vi "EMBL Objective Lock.vi"() -> ()   [LabVIEW 2016]
uses:
  Hardware Configuration/Hardware Configuration Controls/Device Type.ctl
  Hardware Configuration/Hardware Configuration Controls/Device Function.ctl
  Device Library/Cameras/IDS/IDS Controls/IDS Actions.ctl
  Device Library/Stages/Stages Controls/Stage Actions.ctl
  <vilib>/addons/control/pid/pid.llb/PID (DBL Array).vi
  <vilib>/addons/control/pid/NI_PID_pid.lvlib
panel:
  in  "Invert Y":bool
  in  "Invert X":bool
  in  "Flip XY":bool=TRUE
  out "Z Moving":bool
  out "XY Moving":bool
  in  "Lock Z":bool
  in  "Lock Obectives":bool
  in  "Set Lock Position":bool
  in  "Frames Accums":u16=10
  out "Lock Position":dbl[](array[numeric])=[25.486084426867002, 23.515775149080227, -0.6325794284348785]
  out "Current XYZ Positions":dbl[](array[numeric])=[25.44687943773384, 23.028592568780166, -0.15399804743769252]
  out "Difference":dbl[](array[numeric])=[-1.1037470842083863, -0.0443794761167986, 0.0]
  out "Drift Detected":bool
  in  "Z Tolorence":dbl=0.1 format="%#_6f"
  in  "XY Tolorence":dbl=0.1
  out "Z Position":dbl(graph)=-0.15399804743769252
  in  "Display time (ms)":u32=20
  out "Refresh rate":dbl=1.996007984031936
  out "XY Positions":cluster{dbl, dbl}(graph)={25.44687943773384, 23.028592568780166}
  out "ROI":u16[][](graph)=[[103, 104, 97, 86, 80, 79, 59, 70, 55, 56, 44, 54, 47, 62, 70, 96, 116, 143, 146, 167, 194, 216, 232, 243, 276, 307, 316, 310, 318, 306, 280, 274, 267, 251, 222, 199, 175, 157, 125, 107, 87, 79, 57, 56, 38, 36, 28, 30, 24, 26], [123, 104, 98, 92, 87, 76, 65, 64, 66, 52, 69, 62, 71, 73, 96, 114, 138, 166, 199, 194, 218, 242, 260, 295, 331, 342, 361, 346, 350, 340, 317, 299, 293, 261, 252, 217, 194, 165, 145, 128, 105, 87, 76, 51, 48, 30, 28, 22, 28, 24], [122, 120, 100, 101, 92, 83, 72, 80, 72, 75, 78, 75, 87, 106, 115, 133, 161, 204, 233, 237, 264, 308, 326, 347, 361, 372, 377, 375, 398, 398, 373, 345, 325, 304, 289, 250, 222, 195, 169, 151, 119, 94, 76, 64, 40, 34, 26, 22, 20, 40], [145, 128, 110, 114, 100, 92, 88, 78, 84, 89, 95, 101, 121, 132, 142, 159, 213, 251, 284, 298, 327, 380, 398, 409, 441, 433, 455, 453, 443, 443, 422, 397, 394, 352, 342, 288, 269, 231, 203, 175, 145, 113, 98, 62, 57, 38, 39, 28, 36, 39], [139, 139, 120, 127, 99, 110, 95, 101, 109, 110, 107, 129, 145, 174, 180, 217, 248, 292, 318, 359, 384, 454, 490, 490, 525, 519, 514, 518, 526, 513, 506, 478, 441, 413, 379, 338, 301, 269, 233, 202, 155, 129, 104, 79, 54, 52, 38, 34, 33, 32], [163, 150, 138, 123, 119, 123, 121, 106, 133, 139, 152, 156, 181, 200, 223, 260, 317, 350, 367, 397, 455, 527, 570, 568, 603, 588, 628, 616, 635, 622, 594, 550, 534, 480, 451, 387, 350, 312, 264, 215, 187, 145, 125, 93, 78, 57, 44, 45, 40, 34], [167, 162, 159, 145, 130, 141, 127, 137, 147, 161, 172, 202, 214, 237, 271, 330, 391, 414, 453, 471, 518, 611, 636, 655, 673, 706, 747, 724, 736, 729, 670, 633, 619, 550, 509, 458, 389, 342, 288, 252, 199, 172, 145, 117, 98, 78, 59, 53, 44, 46], [189, 174, 175, 161, 162, 150, 154, 165, 176, 192, 217, 254, 269, 282, 330, 382, 460, 502, 550, 586, 631, 694, 719, 759, 772, 816, 837, 848, 825, 831, 774, 709, 675, 607, 560, 490, 454, 380, 334, 280, 241, 200, 165, 133, 117, 87, 72, 62, 58, 56], [189, 194, 182, 181, 174, 173, 171, 197, 200, 212, 243, 300, 316, 352, 386, 460, 509, 577, 651, 704, 737, 784, 823, 844, 891, 920, 949, 942, 941, 922, 849, 810, 743, 672, 617, 545, 500, 436, 383, 336, 276, 243, 195, 159, 129, 117, 91, 85, 70, 67], [212, 214, 200, 185, 208, 193, 200, 218, 239, 254, 305, 348, 365, 409, 482, 511, 595, 660, 739, 790, 846, 925, 944, 985, 1009, 1050, 1073, 1057, 1035, 1038, 958, 864, 842, 773, 705, 631, 589, 518, 444, 385, 312, 261, 231, 181, 167, 132, 114, 105, 93, 78], [217, 227, 216, 221, 229, 216, 224, 260, 270, 310, 355, 382, 414, 478, 553, 613, 668, 765, 847, 907, 965, 1016, 1068, 1109, 1144, 1210, 1225, 1196, 1155, 1130, 1084, 1019, 966, 875, 836, 732, 645, 589, 505, 449, 365, 309, 253, 213, 183, 157, 133, 132, 102, 101], [238, 243, 222, 231, 239, 247, 267, 294, 308, 358, 414, 446, 479, 541, 622, 689, 811, 874, 960, 1009, 1044, 1134, 1223, 1235, 1341, 1337, 1371, 1347, 1340, 1318, 1197, 1152, 1049, 986, 950, 818, 749, 636, 571, 490, 413, 357, 306, 248, 213, 179, 155, 144, 137, 113], [255, 255, 243, 253, 247, 265, 299, 330, 343, 398, 467, 506, 544, 628, 709, 808, 881, 971, 1090, 1152, 1188, 1262, 1309, 1366, 1443, 1501, 1426, 1450, 1425, 1386, 1315, 1221, 1199, 1102, 1011, 902, 816, 728, 642, 554, 484, 410, 354, 297, 252, 222, 178, 165, 154, 143], [256, 252, 253, 273, 281, 290, 340, 355, 389, 439, 517, 547, 608, 697, 814, 877, 967, 1099, 1208, 1299, 1324, 1416, 1427, 1531, 1599, 1607, 1620, 1563, 1556, 1493, 1437, 1362, 1277, 1187, 1093, 991, 922, 815, 721, 627, 541, 490, 386, 338, 282, 241, 222, 197, 187, 160], [269, 283, 273, 300, 302, 316, 365, 389, 441, 506, 554, 594, 684, 794, 899, 995, 1052, 1168, 1286, 1349, 1448, 1558, 1587, 1670, 1742, 1762, 1719, 1716, 1679, 1597, 1517, 1449, 1429, 1313, 1239, 1096, 985, 938, 800, 705, 603, 518, 442, 379, 329, 283, 244, 234, 203, 197], [290, 293, 287, 314, 322, 353, 404, 423, 476, 538, 607, 643, 714, 841, 980, 1084, 1190, 1288, 1381, 1496, 1596, 1625, 1712, 1802, 1901, 1923, 1864, 1865, 1796, 1795, 1654, 1567, 1540, 1396, 1346, 1218, 1132, 957, 879, 773, 667, 577, 492, 418, 352, 307, 274, 243, 241, 211], [295, 310, 309, 343, 344, 381, 431, 475, 505, 566, 667, 706, 793, 914, 1042, 1173, 1301, 1388, 1502, 1657, 1693, 1753, 1789, 1942, 1994, 2031, 1984, 2006, 1939, 1872, 1762, 1653, 1593, 1497, 1410, 1262, 1165, 1022, 927, 813, 683, 632, 545, 452, 391, 356, 296, 272, 253, 243], [322, 320, 327, 356, 370, 408, 458, 505, 547, 596, 680, 732, 874, 1003, 1103, 1207, 1342, 1466, 1617, 1729, 1812, 1865, 1945, 2030, 2069, 2048, 2066, 2075, 2044, 1935, 1828, 1739, 1715, 1563, 1495, 1327, 1214, 1118, 990, 889, 773, 665, 565, 492, 429, 384, 336, 318, 282, 264], [322, 340, 336, 379, 396, 427, 466, 526, 551, 655, 717, 786, 913, 1093, 1189, 1285, 1394, 1566, 1699, 1814, 1892, 1998, 2065, 2147, 2195, 2182, 2206, 2162, 2124, 2065, 1962, 1865, 1793, 1645, 1595, 1427, 1305, 1175, 1051, 909, 810, 690, 603, 545, 456, 408, 366, 333, 308, 281], [332, 343, 355, 389, 409, 441, 487, 506, 576, 658, 778, 849, 966, 1129, 1229, 1342, 1478, 1619, 1781, 1865, 1942, 2021, 2128, 2217, 2270, 2295, 2300, 2280, 2154, 2146, 2027, 1923, 1855, 1712, 1638, 1482, 1338, 1197, 1086, 941, 845, 736, 646, 554, 500, 431, 397, 353, 352, 305], [324, 350, 352, 394, 420, 441, 499, 537, 589, 697, 802, 898, 1009, 1146, 1310, 1345, 1516, 1664, 1848, 1994, 2007, 2120, 2204, 2269, 2301, 2343, 2347, 2332, 2272, 2219, 2085, 1970, 1880, 1743, 1687, 1477, 1341, 1240, 1140, 990, 870, 758, 658, 593, 519, 465, 421, 385, 364, 327], [325, 344, 347, 388, 405, 426, 494, 552, 618, 707, 828, 939, 1040, 1173, 1323, 1412, 1570, 1699, 1839, 2004, 2077, 2157, 2294, 2290, 2367, 2359, 2417, 2368, 2293, 2208, 2118, 2025, 1924, 1825, 1699, 1533, 1389, 1265, 1132, 1020, 905, 799, 696, 610, 548, 490, 460, 411, 385, 343], [300, 328, 326, 366, 391, 426, 476, 562, 625, 723, 864, 938, 1026, 1145, 1342, 1501, 1578, 1748, 1866, 2015, 2089, 2226, 2252, 2306, 2387, 2414, 2428, 2400, 2367, 2264, 2171, 2050, 1955, 1810, 1736, 1557, 1428, 1274, 1175, 1043, 918, 824, 708, 662, 571, 524, 461, 435, 381, 355], [293, 311, 331, 349, 383, 420, 499, 591, 644, 722, 849, 930, 1049, 1146, 1345, 1497, 1633, 1704, 1926, 2019, 2153, 2262, 2232, 2313, 2410, 2386, 2460, 2393, 2372, 2289, 2132, 2046, 1917, 1802, 1696, 1551, 1444, 1278, 1201, 1067, 947, 839, 743, 663, 596, 520, 486, 434, 400, 369], [289, 304, 321, 348, 398, 425, 484, 574, 643, 723, 815, 928, 1041, 1168, 1352, 1492, 1629, 1716, 1871, 2033, 2144, 2270, 2274, 2282, 2393, 2320, 2396, 2393, 2377, 2243, 2173, 2010, 1928, 1828, 1686, 1553, 1444, 1313, 1201, 1040, 924, 863, 759, 668, 610, 560, 495, 456, 418, 365], [289, 300, 333, 340, 393, 417, 476, 550, 624, 683, 803, 907, 1022, 1146, 1343, 1474, 1614, 1698, 1823, 1980, 2060, 2168, 2226, 2345, 2332, 2306, 2376, 2439, 2349, 2280, 2206, 2034, 1930, 1797, 1720, 1542, 1425, 1264, 1175, 1031, 949, 847, 759, 673, 594, 552, 504, 452, 406, 380], [278, 302, 314, 331, 358, 417, 458, 514, 584, 655, 765, 914, 1051, 1127, 1277, 1411, 1589, 1717, 1824, 1958, 2060, 2168, 2226, 2248, 2274, 2208, 2320, 2285, 2217, 2187, 2117, 2022, 1907, 1782, 1668, 1489, 1388, 1257, 1166, 1021, 936, 831, 756, 678, 617, 567, 497, 446, 412, 381], [263, 263, 284, 309, 337, 386, 416, 478, 561, 657, 765, 891, 1016, 1109, 1230, 1350, 1538, 1647, 1755, 1867, 1998, 2119, 2201, 2171, 2217, 2220, 2252, 2205, 2185, 2145, 2031, 1937, 1861, 1722, 1666, 1449, 1372, 1251, 1122, 1021, 914, 825, 753, 649, 601, 541, 480, 433, 414, 371], [226, 235, 264, 284, 305, 362, 413, 459, 551, 648, 727, 828, 965, 1084, 1188, 1337, 1498, 1606, 1700, 1782, 1912, 2021, 2109, 2097, 2187, 2116, 2153, 2099, 2116, 2030, 1952, 1824, 1797, 1640, 1555, 1427, 1315, 1204, 1102, 1012, 874, 803, 725, 642, 583, 513, 469, 434, 399, 389], [219, 215, 243, 261, 285, 338, 392, 432, 532, 627, 703, 785, 898, 1017, 1134, 1267, 1418, 1497, 1634, 1742, 1811, 1953, 1954, 2040, 2103, 2065, 2018, 2004, 1961, 1902, 1821, 1756, 1680, 1558, 1491, 1351, 1265, 1124, 1040, 962, 823, 760, 658, 605, 543, 506, 428, 425, 413, 395], [202, 211, 218, 257, 275, 323, 381, 419, 472, 570, 633, 700, 837, 1004, 1109, 1197, 1344, 1444, 1568, 1669, 1677, 1827, 1871, 1959, 2000, 1944, 1967, 1902, 1845, 1803, 1716, 1664, 1575, 1448, 1358, 1227, 1157, 1052, 953, 864, 759, 709, 623, 547, 510, 472, 447, 427, 416, 380], [188, 196, 201, 233, 253, 272, 321, 371, 426, 502, 616, 698, 788, 932, 1046, 1105, 1220, 1334, 1449, 1565, 1618, 1702, 1739, 1796, 1845, 1875, 1858, 1759, 1739, 1708, 1614, 1500, 1458, 1320, 1294, 1141, 1051, 962, 884, 789, 702, 652, 576, 527, 500, 443, 434, 421, 405, 363], [158, 174, 181, 201, 213, 242, 283, 339, 395, 485, 570, 658, 745, 835, 944, 1063, 1148, 1258, 1373, 1465, 1518, 1620, 1634, 1653, 1707, 1751, 1725, 1652, 1627, 1600, 1476, 1400, 1346, 1214, 1165, 1021, 973, 885, 797, 739, 665, 608, 540, 517, 466, 442, 398, 393, 383, 339], [134, 139, 149, 164, 196, 216, 269, 326, 372, 436, 512, 601, 681, 726, 876, 1004, 1081, 1152, 1240, 1336, 1439, 1485, 1522, 1523, 1582, 1548, 1573, 1576, 1518, 1482, 1381, 1311, 1212, 1146, 1083, 968, 891, 794, 748, 670, 617, 567, 508, 466, 454, 409, 375, 359, 345, 332], [125, 123, 139, 146, 169, 212, 223, 283, 332, 374, 440, 524, 614, 701, 790, 902, 1003, 1052, 1133, 1233, 1307, 1359, 1414, 1423, 1432, 1411, 1404, 1415, 1393, 1349, 1304, 1217, 1147, 1021, 991, 882, 819, 764, 676, 625, 569, 519, 460, 433, 410, 370, 334, 334, 312, 318], [111, 107, 130, 126, 151, 171, 197, 236, 290, 340, 388, 462, 570, 637, 718, 789, 895, 921, 1044, 1081, 1153, 1221, 1285, 1299, 1316, 1261, 1289, 1261, 1220, 1218, 1133, 1065, 1026, 955, 883, 821, 747, 662, 627, 554, 523, 474, 421, 386, 373, 338, 326, 316, 318, 293], [94, 95, 90, 117, 116, 148, 167, 199, 254, 314, 359, 414, 503, 563, 646, 677, 797, 879, 963, 999, 1028, 1119, 1123, 1174, 1195, 1203, 1143, 1103, 1071, 1052, 1005, 938, 891, 842, 780, 699, 650, 569, 529, 500, 446, 400, 367, 344, 316, 298, 300, 298, 313, 288], [75, 70, 72, 92, 101, 114, 161, 189, 226, 264, 326, 361, 426, 492, 598, 631, 689, 775, 822, 907, 922, 977, 984, 1025, 1053, 1064, 1043, 994, 966, 927, 860, 813, 778, 688, 663, 589, 547, 497, 446, 407, 374, 339, 324, 309, 300, 285, 294, 283, 284, 272], [62, 73, 60, 85, 85, 111, 129, 161, 180, 221, 268, 326, 369, 425, 506, 577, 604, 657, 736, 830, 823, 867, 877, 899, 906, 892, 907, 883, 853, 838, 772, 719, 677, 615, 572, 529, 487, 430, 399, 369, 340, 314, 298, 288, 267, 263, 272, 248, 243, 248], [61, 54, 50, 60, 74, 81, 97, 124, 158, 186, 230, 287, 342, 365, 427, 479, 549, 582, 617, 695, 711, 746, 804, 776, 794, 796, 763, 753, 743, 723, 678, 640, 604, 539, 519, 462, 409, 381, 345, 325, 288, 274, 254, 249, 245, 230, 221, 226, 229, 233], [42, 41, 40, 48, 54, 72, 79, 105, 145, 165, 195, 243, 272, 321, 351, 419, 473, 530, 540, 587, 617, 674, 683, 697, 698, 661, 648, 646, 608, 593, 573, 535, 506, 463, 438, 381, 358, 326, 290, 278, 249, 237, 225, 209, 205, 197, 196, 209, 220, 224], [44, 36, 36, 32, 46, 52, 77, 88, 107, 144, 164, 186, 237, 283, 317, 347, 389, 434, 487, 525, 507, 548, 565, 604, 610, 574, 557, 566, 527, 496, 477, 443, 401, 376, 340, 317, 287, 259, 241, 216, 208, 188, 181, 175, 178, 182, 190, 198, 194, 206], [29, 39, 34, 37, 30, 42, 64, 69, 87, 117, 147, 173, 195, 239, 282, 301, 331, 375, 412, 454, 458, 478, 488, 491, 494, 479, 488, 480, 461, 425, 393, 370, 330, 305, 287, 251, 226, 208, 194, 175, 165, 167, 158, 165, 162, 171, 165, 175, 175, 178], [38, 20, 22, 26, 34, 30, 48, 60, 88, 95, 125, 145, 170, 188, 233, 271, 303, 313, 338, 368, 398, 399, 422, 405, 408, 406, 401, 390, 383, 366, 335, 308, 290, 257, 242, 210, 192, 173, 167, 146, 150, 136, 139, 137, 146, 140, 152, 159, 152, 158], [36, 24, 25, 23, 20, 39, 36, 56, 68, 87, 89, 118, 145, 170, 191, 221, 250, 277, 285, 317, 320, 350, 355, 351, 360, 331, 319, 315, 292, 279, 268, 249, 235, 205, 190, 176, 154, 141, 132, 116, 117, 127, 115, 118, 117, 125, 126, 141, 145, 159], [24, 23, 28, 22, 24, 26, 31, 39, 50, 67, 81, 95, 135, 154, 173, 180, 209, 233, 248, 257, 270, 286, 289, 302, 297, 284, 278, 258, 237, 219, 202, 178, 175, 156, 149, 129, 118, 107, 102, 87, 91, 96, 94, 94, 106, 116, 126, 130, 138, 135], [20, 28, 26, 26, 27, 20, 38, 48, 50, 69, 84, 90, 102, 118, 146, 169, 179, 204, 208, 240, 234, 255, 239, 230, 237, 237, 232, 223, 202, 196, 171, 155, 133, 129, 108, 102, 90, 84, 75, 78, 78, 84, 84, 100, 101, 108, 100, 109, 109, 122], [26, 27, 29, 30, 26, 20, 40, 46, 54, 50, 66, 86, 96, 113, 133, 151, 173, 167, 177, 184, 219, 219, 203, 201, 199, 180, 180, 170, 159, 152, 139, 119, 106, 93, 93, 81, 75, 62, 70, 64, 74, 64, 82, 74, 86, 90, 91, 100, 107, 112], [22, 23, 25, 25, 21, 32, 34, 34, 40, 50, 60, 72, 92, 102, 111, 129, 140, 164, 161, 165, 163, 187, 180, 182, 165, 159, 151, 141, 124, 114, 100, 103, 84, 81, 70, 63, 54, 57, 49, 55, 52, 52, 58, 60, 75, 81, 81, 100, 94, 106], [36, 25, 25, 20, 30, 20, 34, 42, 52, 55, 69, 71, 88, 92, 114, 111, 127, 126, 146, 154, 158, 148, 148, 145, 150, 143, 129, 115, 113, 90, 88, 64, 66, 50, 47, 40, 43, 42, 48, 39, 48, 52, 54, 68, 69, 77, 80, 82, 86, 80]]
  in  "ROI Half Width":i32=25
  out "Intensity Graph":u16[][](graph)
  in  "Quit":bool
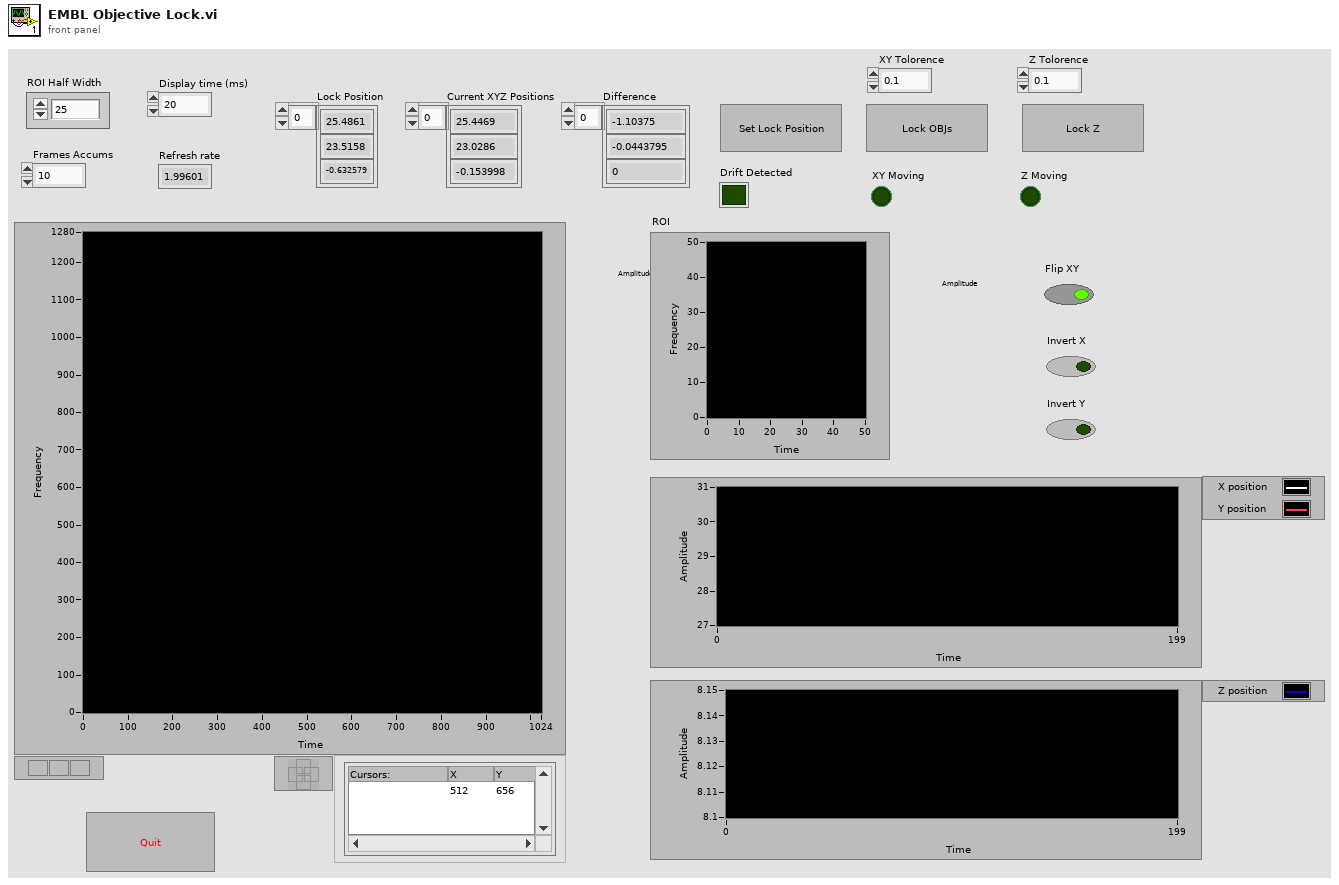
[diagram p1: front panel]
types:
  T1 = typedef "Stage Actions.ctl" = enum16{"Get Position", "MVR", "MOVE", "HALT", "ONTARGET", "ERROR", "REFERENCE", "INIT", "VELOCITY", "STATUS", "EXIT", "HOME", "ZEROPOS", "NANOPOS", "ANALOG", "QUIT"}
  T2 = typedef "IDS Actions.ctl" = enum16{"Error Check", "Initialize", "Preview", "Record", "Abort", "Record Settings", "Set Parameter", "Get Parameter", "Set ROI", "Get ROI", "Status", "Quit"}
  T3 = typedef "Device Function.ctl" = enum16{"Primary", "Secondary", "Overview", "Wide Field Drift Correction", "642 nm Excitation", "560 nm Excitation", "546 nm Excitation", "488 nm Excitation", "405 nm Excitation", "Objective Drift Correction", "4Pi Objective Lock", "Objective XY", "Objective Z", "Sample XY", "Sample Coarse Z", "Sample Z", "4Pi Lower", "4Pi Upper", "Adj Cavity", "Line Scanning", "Alert"}
  T4 = typedef "Device Type.ctl" = enum16{"AOTF", "Camera", "Deformable Mirror", "Laser", "Shutter", "Stage", "Waveform", "Email"}
  T5 = cluster{"proportional gain (Kc)":dbl, "integral time (Ti, min)":dbl, "derivative time (Td, min)":dbl}[]
  T6 = typedef "LVCursorListTypeDef.ctl" = cluster{"Name":string, "Color":u32, "Style":u8, "Point Style":u8, "Name Visible":bool, "Allow Drag":bool, "Cursor Mode":u32, "Plot":i32, "Index":i32, "Position":cluster{"X":dbl, "Y":dbl}, "X Scale":u32, "Y Scale":u32, "Watch Plots":i32[], "Watch All Plots":bool, "Plot Area":i32, "Label Offset":cluster{"X":dbl, "Y":dbl}}[]
  T7 = cluster{"Name":string, "Color":u32, "Style":u8, "Point Style":u8, "Name Visible":bool, "Allow Drag":bool, "Cursor Mode":u32, "Plot":i32, "Index":i32, "Position":cluster{"X":dbl, "Y":dbl}, "X Scale":u32, "Y Scale":u32, "Watch Plots":i32[], "Watch All Plots":bool, "Plot Area":i32, "Label Offset":cluster{"X":dbl, "Y":dbl}}
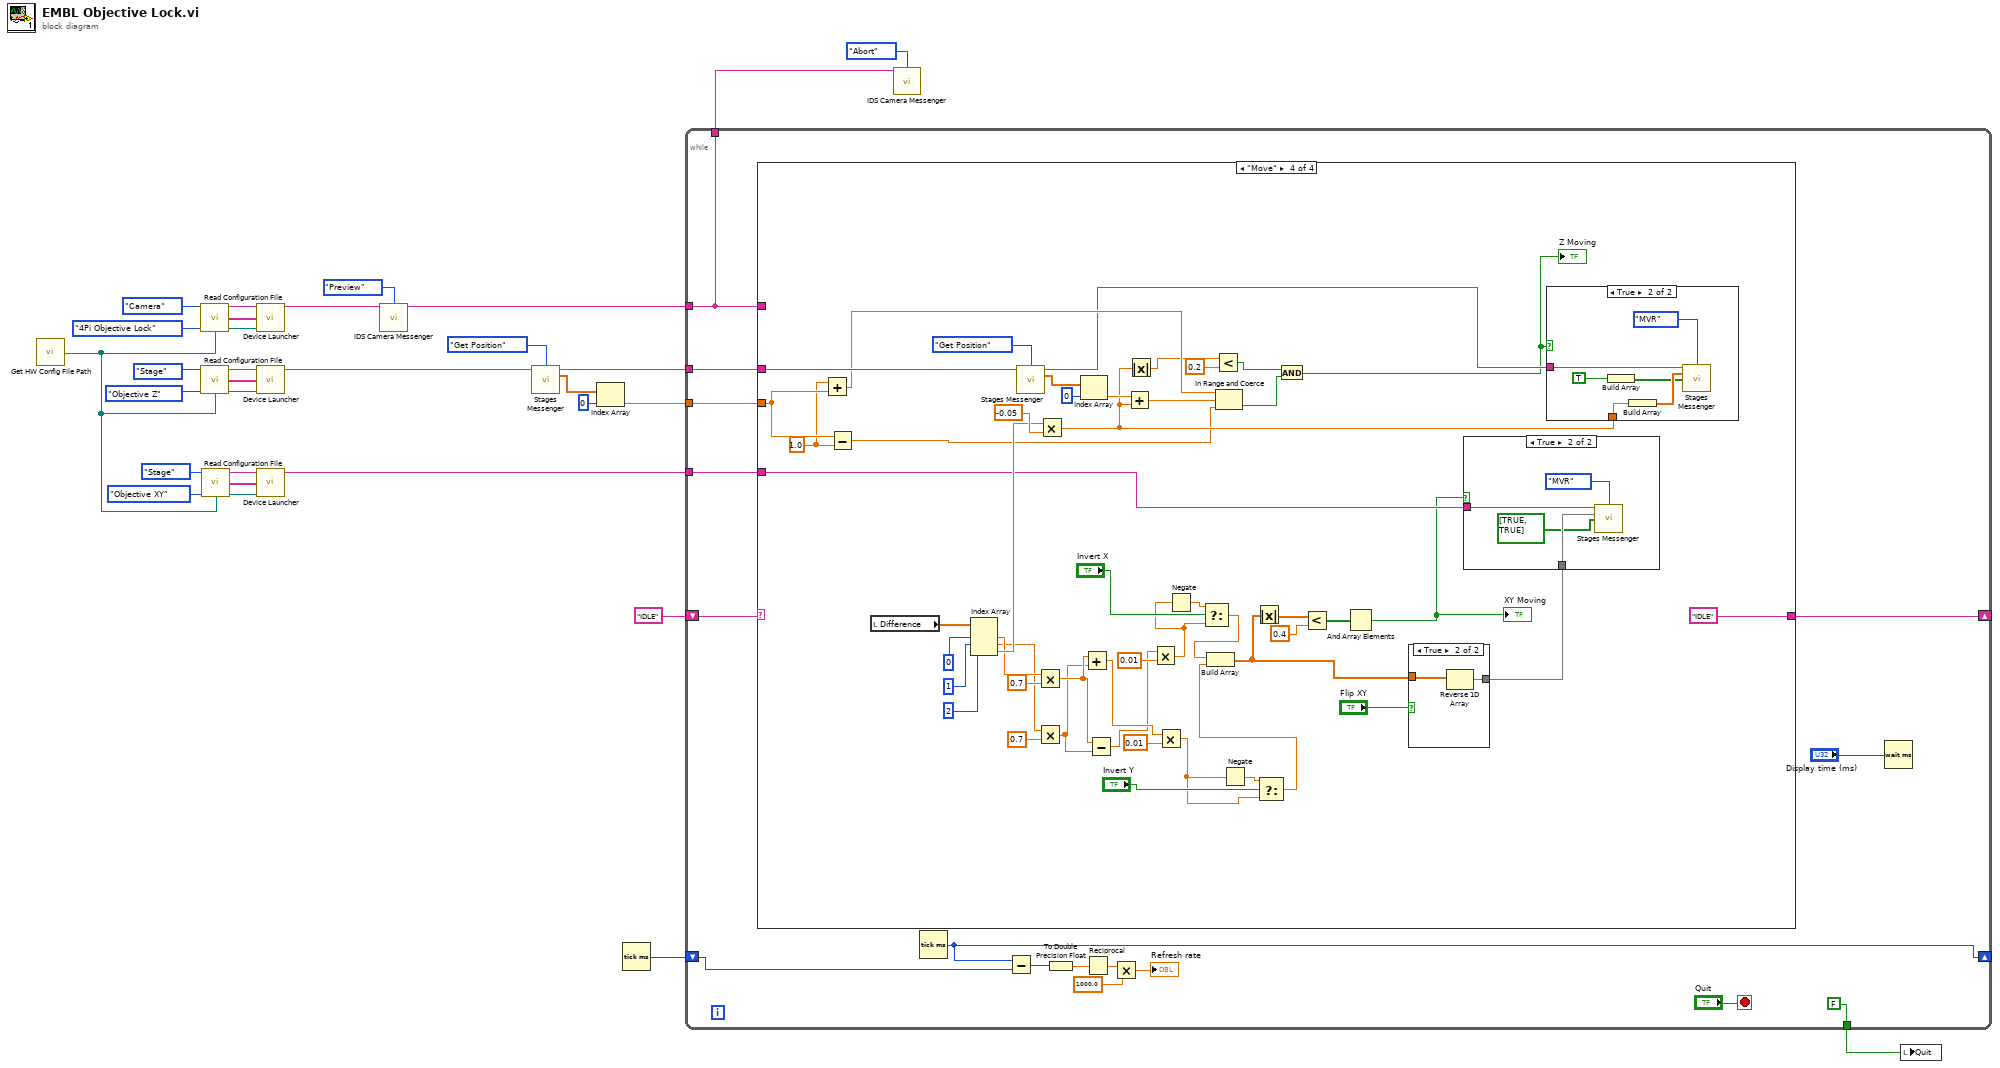
[diagram p0: block diagram]
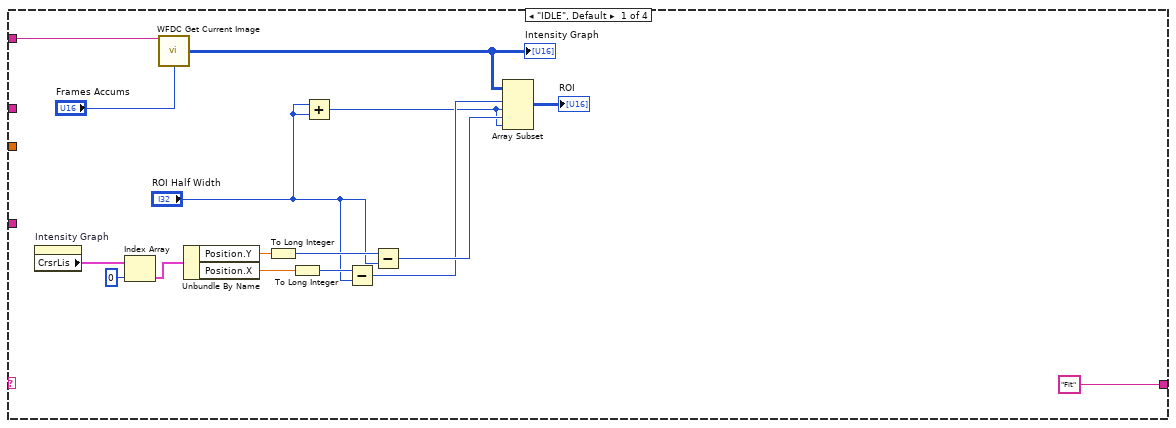
[diagram p2: hidden frame]
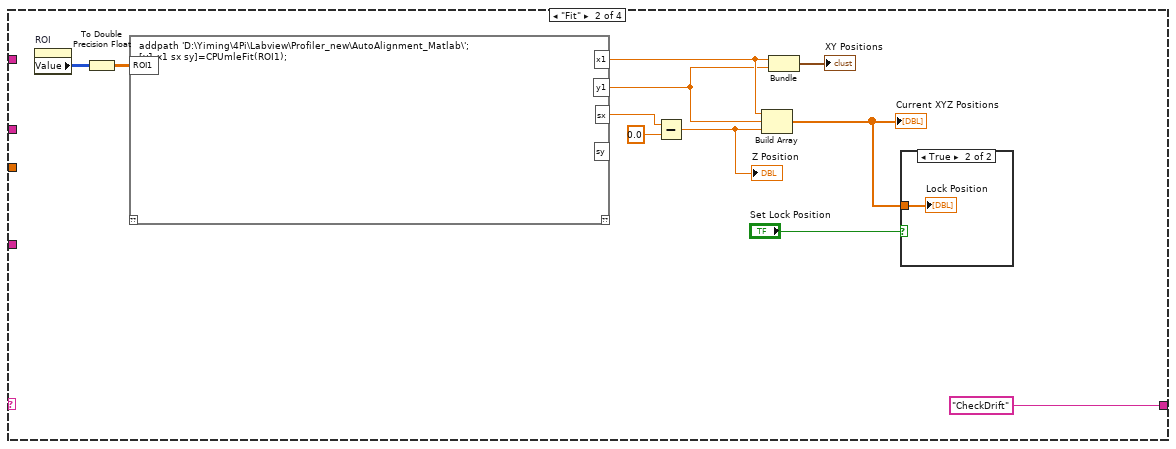
[diagram p3: hidden frame]
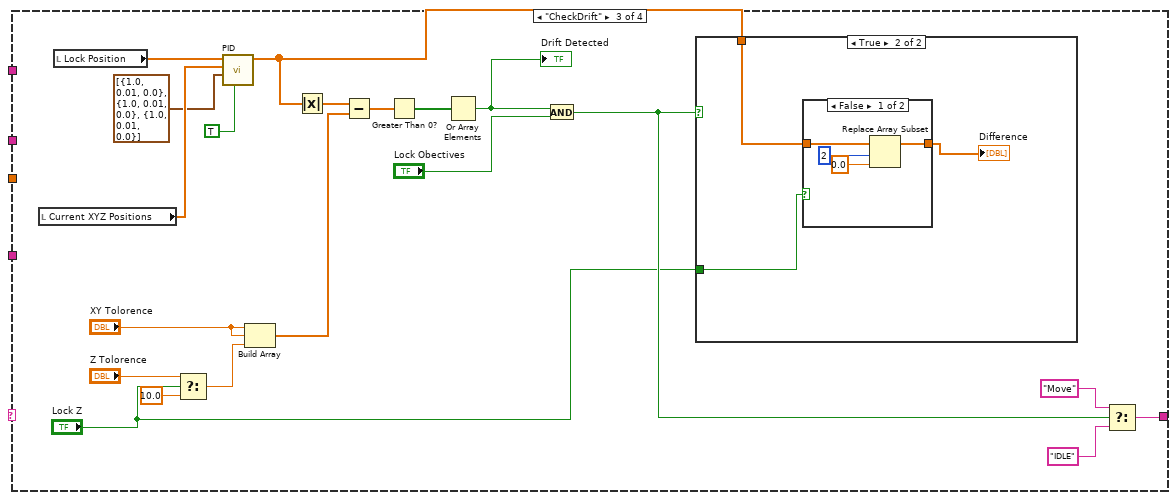
[diagram p5: hidden frame]
diagram:
  n1 = call "Get HW Config File Path.vi"() -> ("File Path"=w14:path)  [unwired: 14 in, 1 out]
  n2 = call "Read Configuration File.vi"("Device Type"=Device_Type."Camera", "Device Function"=Device_Function."4Pi Objective Lock", "Config File Path"=w14) -> ("Unique Notifier Name"=w27:string, "Device Ports/IDs/Channels"=w29:string[], "Device Engine Path"=w28:path)  [unwired: 9 in, 1 out]
  n3 = call "Read Configuration File.vi"("Device Type"=Device_Type."Stage", "Device Function"=Device_Function."Objective Z", "Config File Path"=w14) -> ("Unique Notifier Name"=w22:string, "Device Ports/IDs/Channels"=w20:string[], "Device Engine Path"=w21:path)  [unwired: 9 in, 1 out]
  n4 = call "Read Configuration File.vi"("Device Type"=Device_Type."Stage", "Device Function"=Device_Function."Objective XY", "Config File Path"=w14) -> ("Unique Notifier Name"=w15:string, "Device Ports/IDs/Channels"=w16:string[], "Device Engine Path"=w17:path)  [unwired: 9 in, 1 out]
  n5 = call "Device Launcher.vi"("Notifier Name"=w27, "Device Ports/IDs/Channels"=w29, "Device Engine Path"=w28) -> ("Notifier Name"=w13:string)  [unwired: 11 in, 1 out]
  n6 = call "Device Launcher.vi"("Notifier Name"=w22, "Device Ports/IDs/Channels"=w20, "Device Engine Path"=w21) -> ("Notifier Name"=w7:string)  [unwired: 11 in, 1 out]
  n7 = call "Device Launcher.vi"("Notifier Name"=w15, "Device Ports/IDs/Channels"=w16, "Device Engine Path"=w17) -> ("Notifier Name"=w11:string)  [unwired: 11 in, 1 out]
  n8 = call "IDS Camera Messenger.vi"("Notifier Name"=w13, "IDS Actions"=IDS_Actions."Preview") -> ("Notifier Name (Dup)"=w2:string)  [unwired: 8 in, 5 out]
  n9 = call "Stages Messenger.vi"("Stage Notifier Name"=w7, "Actions"=Stage_Actions."Get Position") -> ("Stage Notifier Name (Dup)"=w6:string, "Positions"=w4:dbl[])  [unwired: 10 in, 2 out]
  n10 = Index Array(array=w4, index=0) -> (element=w3:dbl)
  n11 = Tick Count (ms)() -> (millisecond timer value=w30:u32)
  n12 = while {
    shift-right: [w46] -> _
    shift-left: "IDLE" -> [w47]
    tunnel: w11 -> [w44]
    shift-right: [w42] -> _
    shift-left: w30 -> [w43]
    tunnel: w6 -> [w36]
    tunnel: w2 -> [w34]
    tunnel: [w34] -> w9
    tunnel: w3 -> [w33]
    tunnel: [FALSE] -> w1
    stop <- "Quit" stop-if-true
    n13 = case shown="\"Move\"" w47 {
      tunnel: ["Fit" ("t") "CheckDrift" w79 "IDLE" ("t")] -> w46
      tunnel: w44 -> [_ _ _ w136]
      tunnel: w36 -> [_ _ _ w134]
      tunnel: w34 -> [w62 _ _ _]
      tunnel: w33 -> [_ _ _ w128]
      frame "IDLE", Default {
        n14 = property on="Intensity Graph" class="IntGraph (strict)"() -> ("CrsrLis"=w51:T6)  [unwired: 2 in, 2 out]
        n15 = Index Array(array=w51, index=0) -> (element=w49:T7)
        n16 = call "WFDC Get Current Image.vi"("IDS Camera Notifier Name"=w62, "Frames"="Frames Accums") -> ("Image - U16"=w61:u16[][])  [unwired: 11 in, 2 out]
        "Intensity Graph" <- w61
        n17 = Unbundle By Name(w49) -> ("Position.Y"=w59:dbl, "Position.X"=w58:dbl)
        n18 = To Long Integer(number=w59) -> (32bit integer=w57:i32)
        n19 = To Long Integer(number=w58) -> (32bit integer=w56:i32)
        n20 = Add(x="ROI Half Width", y="ROI Half Width") -> (x+y=w52:i32)
        n21 = Subtract(x=w56, y="ROI Half Width") -> (x-y=w54:i32)
        n22 = Subtract(x=w57, y="ROI Half Width") -> (x-y=w55:i32)
        n23 = Array Subset(array=w61, index (row)=w54, length (row)=w52, index (col)=w55, length (col)=w52) -> (→"ROI":u16[][])
      }
      frame "Fit" {
        n24 = property on="ROI" class="IntGraph (strict)"() -> ("Value"=w73:u16[][])  [unwired: 2 in, 2 out]
        n25 = To Double Precision Float(number=w73) -> (double precision float=w70:dbl[][])
        n26 = script code="addpath 'D:\\Yiming\\4Pi\\Labview\\Profiler_new\\AutoAlignment_Matlab\\';\n[y1 x1 sx sy]=CPUmleFit(ROI1);"("ROI1"=w70) -> ("x1"=w69:dbl, "y1"=w68:dbl, "sx"=w67:dbl)  [unwired: 1 in, 2 out]
        n27 = Subtract(x=w67, y=0.0) -> (x-y=w71:dbl)
        "Z Position" <- w71
        n28 = Build Array(w69, w68, w71) -> (w64:dbl[])
        "Current XYZ Positions" <- w64
        n29 = Bundle(w69, w68) -> (→"XY Positions":cluster{dbl, dbl})  [unwired: 1 in]
        n30 = case shown="True" "Set Lock Position" {
          tunnel: w64 -> [_ w75]
          frame False {
          }
          frame True {
            "Lock Position" <- w75
          }
        }
      }
      frame "CheckDrift" {
        n31 = local read "Current XYZ Positions"() -> (w86:dbl[])
        n32 = local read "Lock Position"() -> (w87:dbl[])
        n33 = Select(t="Z Tolorence", s="Lock Z", f=10.0) -> (s? t:f=w88:dbl)
        n34 = call-poly <vilib>:"PID.vi"("reinitialize? (F)"=TRUE, "PID gains"=T5 [{"proportional gain (Kc)"=1.0, "integral time (Ti, min)"=0.01, "derivative time (Td, min)"=0.0}, {"proportional gain (Kc)"=1.0, "integral time (Ti, min)"=0.01, "derivative time (Td, min)"=0.0}, {"proportional gain (Kc)"=1.0, "integral time (Ti, min)"=0.01, "derivative time (Td, min)"=0.0}], "process variable"=w86, "setpoint"=w87) -> ("output"=w77:dbl[])  [unwired: 6 in, 1 out]
        n35 = Build Array("XY Tolorence", "XY Tolorence", w88) -> (w78:dbl[])
        n36 = Absolute Value(x=w77) -> (abs(x)=w94:dbl[])
        n37 = Subtract(x=w94, y=w78) -> (x-y=w92:dbl[])
        n38 = Greater Than 0?(x=w92) -> (x > 0?=w93:bool[])
        n39 = Or Array Elements(Boolean array=w93) -> (logical OR=w91:bool)
        "Drift Detected" <- w91
        n40 = And(x=w91, y="Lock Obectives") -> (x .and. y?=w80:bool)
        n41 = case shown="True" w80 {
          tunnel: w77 -> [_ w98]
          tunnel: "Lock Z" -> [_ w96]
          frame False {
          }
          frame True {
            n42 = case shown="False" w96 {
              tunnel: w98 -> [w100 w103]
              tunnel: [w99 w103] -> w97
              frame False {
                n43 = Replace Array Subset(array=w100, new element=0.0 ("new element/subarray"), index=2) -> (w99:dbl[])
              }
              frame True {
              }
            }
            "Difference" <- w97
          }
        }
        n44 = Select(t="Move", s=w80, f="IDLE") -> (s? t:f=w79:string)
      }
      frame "Move" {
        w127 = 1.0 ("y")
        n45 = Add(x=w127, y=w128) -> (x+y=w126:dbl)
        n46 = Subtract(x=w128, y=w127) -> (x-y=w125:dbl)
        n47 = local read "Difference"() -> (w151:dbl[])
        n48 = Index Array(array=w151, index #1=0 ("index"), index #2=1 ("index"), index #3=2 ("index")) -> (element #1=w144:dbl, element #2=w141:dbl, element #3=w147:dbl)
        n49 = call "Stages Messenger.vi"("Stage Notifier Name"=w134, "Actions"=Stage_Actions."Get Position") -> ("Stage Notifier Name (Dup)"=w117:string, "Positions"=w133:dbl[])  [unwired: 10 in, 2 out]
        n50 = Multiply(x=w144, y=0.7) -> (x*y=w140:dbl)
        n51 = Multiply(x=w141, y=0.7) -> (x*y=w139:dbl)
        n52 = Multiply(x=w147, y=-0.05) -> (x*y=w130:dbl)
        n53 = Index Array(array=w133, index=0) -> (element=w131:dbl)
        n54 = Add(x=w140, y=w139) -> (x+y=w138:dbl)
        n55 = Subtract(x=w140, y=w139) -> (x-y=w137:dbl)
        n56 = Add(x=w131, y=w130) -> (x+y=w129:dbl)
        n57 = Absolute Value(x=w130) -> (abs(x)=w124:dbl)
        n58 = Multiply(x=w137, y=0.01) -> (x*y=w109:dbl)
        n59 = Multiply(x=w138, y=0.01) -> (x*y=w105:dbl)
        n60 = Negate(x=w109) -> (-x=w110:dbl)
        n61 = Select(t=w110, s="Invert X", f=w109) -> (s? t:f=w108:dbl)
        n62 = Less?(x=w124, y=0.2) -> (x < y?=w122:bool)
        n63 = In Range and Coerce(upper limit=w126, x=w129, lower limit=w125) -> (In Range?=w121:bool)  [unwired: 1 out]
        n64 = Negate(x=w105) -> (-x=w107:dbl)
        n65 = Select(t=w107, s="Invert Y", f=w105) -> (s? t:f=w104:dbl)
        n66 = Build Array(w108, w104) -> (w113:dbl[])
        n67 = Absolute Value(x=w113) -> (abs(x)=w120:dbl[])
        n68 = And(x=w122, y=w121) -> (x .and. y?=w116:bool)
        "Z Moving" <- w116
        n69 = Less?(x=w120, y=0.4) -> (x < y?=w118:bool[])
        n70 = And Array Elements(Boolean array=w118) -> (logical AND=w115:bool)
        "XY Moving" <- w115
        n71 = case shown="True" "Flip XY" {
          tunnel: w113 -> [w154 w156]
          tunnel: [w154 w155] -> w112
          frame False {
          }
          frame True {
            n72 = Reverse 1D Array(array=w156) -> (reversed array=w155:dbl[])
          }
        }
        n73 = case shown="True" w115 {
          tunnel: w136 -> [_ w160]
          tunnel: w112 -> [_ w159]
          frame False {
          }
          frame True {
            n74 = call "Stages Messenger.vi"("Stage Notifier Name"=w160, "Actions"=Stage_Actions."MVR", "Setpoint"=w159, "Axis"=bool[] [TRUE, TRUE]) -> ()  [unwired: 8 in, 4 out]
          }
        }
        n75 = case shown="True" w116 {
          tunnel: w130 -> [_ w162]
          tunnel: w117 -> [_ w161]
          frame False {
          }
          frame True {
            n76 = Build Array(TRUE) -> (w164:bool[])
            n77 = Build Array(w162) -> (w165:dbl[])
            n78 = call "Stages Messenger.vi"("Stage Notifier Name"=w161, "Actions"=Stage_Actions."MVR", "Setpoint"=w165, "Axis"=w164) -> ()  [unwired: 8 in, 4 out]
          }
        }
      }
    }
    n79 = Tick Count (ms)() -> (millisecond timer value=w42:u32)
    n80 = Subtract(x=w42, y=w43) -> (x-y=w41:u32)
    n81 = To Double Precision Float(number=w41) -> (double precision float=w40:dbl)
    n82 = Reciprocal(x=w40) -> (1/x=w39:dbl)
    n83 = Multiply(x=w39, y=1000.0) -> (x*y=→"Refresh rate":dbl)
    n84 = Wait (ms)(milliseconds to wait="Display time (ms)") -> ()  [unwired: 1 out]
  }
  n85 = call "IDS Camera Messenger.vi"("Notifier Name"=w9, "IDS Actions"=IDS_Actions."Abort") -> ()  [unwired: 8 in, 6 out]
  n86 = local write "Quit"(w1) -> ()
